vi "LoadWave.vi"(10 "Variables":T3={"Number of rings"=1, "sound spd (cm/s)"=150000, "z span (cm)"=4.0, "z steps"=20, "y spacing (cm)"=0.01, "y steps"=50, "time step (s)"=1e-08, "z"=0.0, "y"=0.0, "ref delay"=0.0, "freq (MHz)"=4.71, "cycles"=300.0} {"freq (MHz)" format="%.2f"; "z span (cm)" format="%.2f"; "y" format="%.2f"; "ref delay" format="%.2f"; "y spacing (cm)" format="%.2f"; "z" format="%.2f"; "time step (s)" format="%.2e"}, 11 "Wave Source":T1={"Load Wave File"=FALSE, "file path"=path "F:/PVDFXducer/FiveRing/5Ring5/83micH/R1quartz.txt", "Up sample fac"=1}) -> (3 "Waveform Graph":dbl[](graph))   [LabVIEW 2022 SP3]
uses:
  <vilib>/Analysis/4window.llb/Hamming Window (DBL).vi
  <vilib>/Analysis/4window.llb/AllCosWindow (DBL).vi
  <vilib>/Utility/file.llb/Read From Spreadsheet File (DBL).vi
  <vilib>/Analysis/2dsp.llb/Rational Resample (single channel, DBL).vi
  <vilib>/Analysis/NI_AALPro.lvlib
panel:
  out "Spectrum":T2(graph)
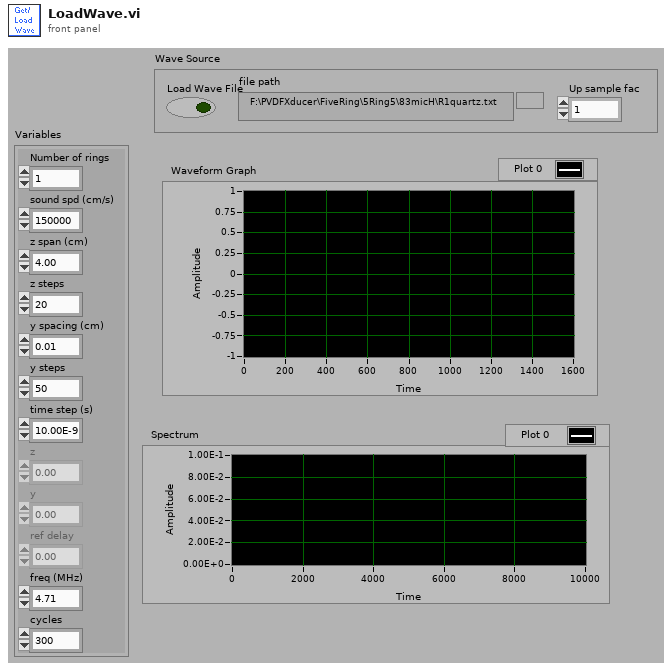
[diagram p1: front panel]
types:
  T1 = cluster{"Load Wave File":bool, "file path":path, "Up sample fac":i32}
  T2 = cluster{i32, "df":dbl, "Power Spectrum (V^2 rms)":dbl[]}
  T3 = cluster{"Number of rings":i32, "sound spd (cm/s)":i32, "z span (cm)":dbl, "z steps":i32, "y spacing (cm)":dbl, "y steps":i32, "time step (s)":sgl, "z":dbl, "y":dbl, "ref delay":dbl, "freq (MHz)":dbl, "cycles":sgl}
  T4 = enum16{"sine", "cosine", "triangle", "square", "sawtooth", "increasing ramp", "decreasing ramp"}
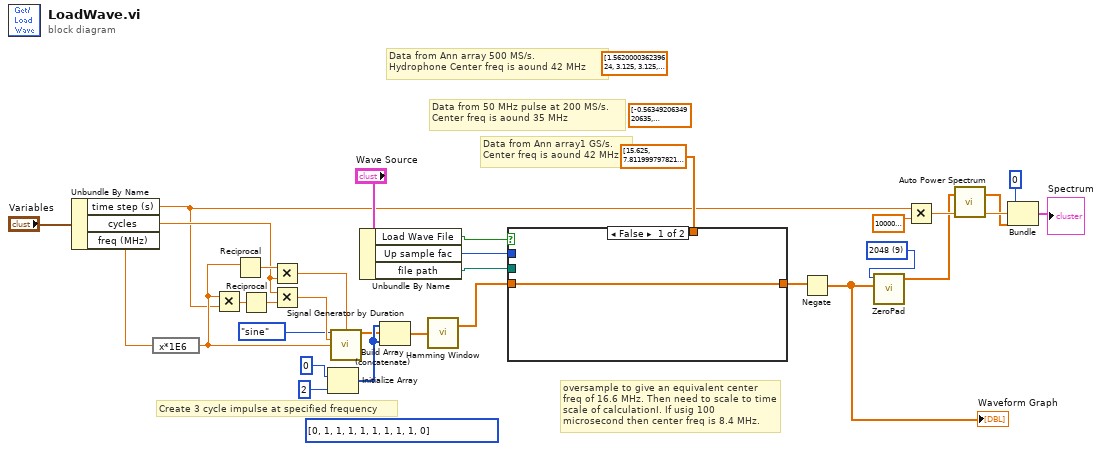
[diagram p0: block diagram]
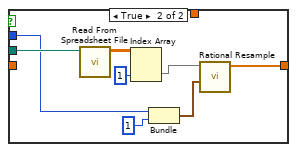
[diagram p2: hidden frame]
diagram:
  w2 = u16 9 items=["next 2^n", "8", "16", "32", "64", "128", "256", "512", "1024", "2048"] ("FFT size")
  (unwired) sgl[] [1.562, 3.125, 3.125, 3.906, 3.125, 1.562, 1.562, 2.344, 3.125, 3.125, 3.125, 3.906, 4.687, 4.687, 5.469, 4.687, 3.125, 1.562, 1.562, 0.781, 1.562, 1.562, 1.562, 3.125, 3.125, 2.344, 1.562, 3.125, 2.344, 0.781, 0.0, 0.0, -0.781, -0.781, 0.0, 1.562, 3.125, 3.125, 3.125, 3.125, 2.344, 1.562, -0.781, -0.781, 0.781, 3.125, 3.125, 3.906, 3.906, 3.906, 4.687, 3.125, 1.562, 1.562, 2.344, 2.344, 2.344, 3.125, 3.906, 3.125, 2.344, 0.781, 0.0, -0.781, 0.781, 0.781, 0.781, 0.781, 0.781, 0.0, 0.0, 0.0, 0.0, 0.0, -0.781, -1.562, -3.125, -3.125, -4.687, -3.906, -7.031, -10.156, -12.5, -16.406, -18.75, -22.656, -24.219, -18.75, -9.375, 7.812, 28.125, 47.656, 65.625, 73.437, 73.437, 66.406, 53.906, 41.406, 27.344, 14.844, 3.906, -5.469, -14.062, -22.656, -25.781, -26.562, -25.0, -24.219, -21.875, -21.875, -25.0, -28.125, -32.812, -37.5, -44.531, -46.875, -43.75, -32.031, -15.625, 3.125, 25.0, 39.062, 47.656, 50.0, 45.312, 35.156, 24.219, 13.281, 4.687, -3.906, -9.375, -12.5, -13.281, -17.187, -17.187, -14.062, -7.812, -3.125, 1.562, 0.781, -0.781, -3.906, -6.25, -8.594, -8.594, -9.375, -7.031, -3.125, 0.0, 4.687, 6.25, 8.594, 8.594, 10.937, 10.156, 10.156, 9.375, 7.812, 4.687, 1.562, -0.781, -2.344, -3.125, -3.906, -3.125, -2.344, -0.781, 1.562, 3.125, 3.125, 1.562, 1.562, 1.562, 1.562, 1.562, 2.344, 3.906, 3.125, 3.125, 3.125, 2.344, 2.344, 0.781, -0.781, 0.0, 3.125, 4.687, 6.25, 5.469, 5.469, 6.25, 6.25, 6.25, 4.687, 6.25, 7.031, 6.25, 6.25, 6.25, 9.375, 9.375, 7.812, 7.031, 7.031, 7.031, 5.469, 5.469, 5.469, 5.469, 5.469, 4.687, 3.125, 3.125, 2.344, 2.344, 1.562, 3.125, 5.469, 5.469, 5.469, 5.469, 5.469, 5.469, 4.687, 3.906, 3.906, 3.125, 3.125, 3.906, 2.344, 1.562, 2.344, 2.344, 3.125, 3.125, 3.125, 3.125, 3.125, 1.562, 0.781, 0.0, 0.781, 0.0] ("first row")
  (unwired) i32[] [0, 1, 1, 1, 1, 1, 1, 1, 1, 0] ("first row")
  (unwired) dbl[] [-0.5634920634920635, -0.6825396825396826, -0.8015873015873016, -0.9920634920634921, -1.1507936507936507, -1.3888888888888888, -1.992063492063492, -4.2063492063492065, -5.888888888888889, 13.023809523809524, 61.32539682539682, 92.83333333333333, 75.10317460317461, 18.126984126984127, -54.93650793650794, -109.60317460317461, -104.22222222222223, 18.134920634920636, 83.33333333333333, 27.27777777777778, -42.19047619047619, -45.63492063492063, 10.15079365079365, 49.05555555555556, 28.19047619047619, -5.658730158730159, -15.261904761904763, -4.4603174603174605, 7.984126984126984, 10.682539682539682, 5.809523809523809, -0.03968253968253968, -2.515873015873016, -1.4841269841269842, 1.0396825396825398, 2.0555555555555554, 0.9523809523809523, -0.6031746031746031, -1.007936507936508, -0.3968253968253968, 0.14285714285714285] ("Array")
  # "Create 3 cycle impulse at specified frequency"
  # "Data from Ann array 500 MS/s.\nHydrophone Center freq is aound 42 MHz"
  # "Data from Ann array1 GS/s.\nCenter freq is aound 42 MHz"
  # "oversample to give an equivalent center freq of 16.6 MHz. Then need to scale to time scale of calculationI. If usig 100 microsecond then center freq is 8.4 MHz."
  # "Data from 50 MHz pulse at 200 MS/s.\nCenter freq is aound 35 MHz"
  n1 = Unbundle By Name("Variables") -> ("time step (s)"=w5:sgl, "cycles"=w19:sgl, "freq (MHz)"=w20:dbl)
  n2 = expression code="x*1E6"(w20) -> (w23:dbl)
  n3 = Multiply(x=w23, y=w5) -> (x*y=w27:dbl)
  n4 = Reciprocal(x=w23) -> (1/x=w22:dbl)
  n5 = Reciprocal(x=w27) -> (1/x=w24:dbl)
  n6 = Multiply(x=w22, y=w19) -> (x*y=w21:dbl)
  n7 = Multiply(x=w19, y=w24) -> (x*y=w26:dbl)
  n8 = Initialize Array(0, 2) -> (w16:i32[])
  n9 = call <vilib>:"Signal Generator by Duration.vi"("signal type"=T4."sine", "duration"=w21, "# of samples"=w26, "frequency"=w23) -> ("signal"=w15:dbl[])  [unwired: 3 in, 8 out]
  n10 = Unbundle By Name("Wave Source") -> ("Load Wave File"=w11:bool, "Up sample fac"=w10:i32, "file path"=w9:path)
  n11 = Build Array (concatenate)(w16, w15, w16) -> (w8:dbl[])
  n12 = call-poly <vilib>:"Hamming Window.vi"("X"=w8) -> ("Windowed X"=w7:dbl[])  [unwired: 1 out]
  n13 = case shown="False" w11 {
    tunnel: [w33 w35] -> w4
    tunnel: w7 -> [w33 _]
    tunnel: w9 -> [_ w39]
    tunnel: w10 -> [_ w37]
    tunnel: sgl[] [15.625, 7.812, 7.812, 7.812, 0.0, 7.812, 7.812, 0.0, 0.0, 7.812, 7.812, 7.812, 7.812, 7.812, 7.812, 7.812, 7.812, 7.812, 7.812, 15.625, 7.812, 7.812, 7.812, 15.625, 7.812, 7.812, 7.812, 7.812, 7.812, 15.625, 7.812, 7.812, 7.812, 7.812, 7.812, 7.812, 7.812, 0.0, 7.812, 7.812, 7.812, 0.0, 0.0, 7.812, 7.812, 7.812, 0.0, 7.812, 7.812, 7.812, 7.812, 7.812, 7.812, 7.812, 15.625, 7.812, 7.812, 7.812, 7.812, 7.812, 7.812, 7.812, 7.812, 7.812, 7.812, 7.812, 7.812, 7.812, 7.812, 0.0, 7.812, 7.812, 7.812, 15.625, 7.812, 7.812, 7.812, 7.812, 15.625, 7.812, 7.812, 15.625, 7.812, 7.812, 7.812, 15.625, 0.0, 7.812, 15.625, 7.812, 15.625, 7.812, 7.812, 7.812, 7.812, 7.812, 0.0, 7.812, 7.812, 7.812, 7.812, 7.812, 7.812, 7.812, 7.812, 7.812, 7.812, 7.812, 15.625, 7.812, 7.812, 7.812, 7.812, 7.812, 15.625, 7.812, 7.812, 7.812, 7.812, 7.812, 7.812, 7.812, 7.812, 0.0, 7.812, 0.0, 7.812, 7.812, 7.812, 7.812, 7.812, 7.812, 7.812, 7.812, 7.812, 7.812, 7.812, 7.812, 7.812, 7.812, 0.0, 15.625, 0.0, 7.812, 7.812, 7.812, 7.812, 15.625, 15.625, 7.812, 7.812, 7.812, 7.812, 7.812, 7.812, 7.812, 7.812, 7.812, 7.812, 7.812, 7.812, 7.812, 7.812, 7.812, 7.812, 7.812, 7.812, 7.812, 7.812, 7.812, 15.625, 15.625, 7.812, 7.812, 7.812, 7.812, 0.0, 0.0, 0.0, 7.812, 7.812, 7.812, 7.812, 0.0, 7.812, 15.625, 7.812, 7.812, 15.625, 7.812, 15.625, 7.812, 7.812, 7.812, 7.812, 7.812, 7.812, 7.812, 15.625, 7.812, 7.812, 7.812, 7.812, 7.812, 15.625, 7.812, 7.812, 7.812, 7.812, 7.812, 7.812, 7.812, 7.812, 15.625, 7.812, 7.812, 15.625, 7.812, 15.625, 7.812, 7.812, 7.812, 7.812, 7.812, 7.812, 7.812, 15.625, 15.625, 7.812, 7.812, 7.812, 7.812, 7.812, 15.625, 7.812, 7.812, 7.812, 7.812, 7.812, 7.812, 7.812, 7.812, 7.812, 7.812, 0.0, 7.812, 0.0, 0.0, 7.812, 15.625, 7.812, 7.812, 7.812, 7.812, 7.812, 7.812, 7.812, 7.812, 7.812, 7.812, 7.812, 15.625, 7.812, 7.812, 7.812, 7.812, 7.812, 0.0, 7.812, 7.812, 7.812, 7.812, 7.812, 7.812, 0.0, 0.0, 7.812, 7.812, 7.812, 0.0, 7.812, 7.812, 7.812, 7.812, 7.812, 7.812, 7.812, 7.812, 15.625, 7.812, 7.812, 15.625, 7.812, 7.812, 7.812, 7.812, 7.812, 7.812, 0.0, 7.812, 7.812, 7.812, 15.625, 7.812, 7.812, 7.812, 7.812, 7.812, 7.812, 7.812, 7.812, 7.812, 7.812, 15.625, 7.812, 7.812, 7.812, 7.812, 7.812, 0.0, 7.812, 7.812, 7.812, 7.812, 7.812, 7.812, 7.812, 7.812, 7.812, 15.625, 15.625, 7.812, 7.812, 7.812, 0.0, 7.812, 7.812, 7.812, 7.812, 7.812, 7.812, 7.812, 0.0, 7.812, 7.812, 7.812, 7.812, 7.812, 7.812, 7.812, 0.0, 7.812, 0.0, 7.812, 15.625, 7.812, 7.812, 7.812, 0.0, 7.812, 7.812, 7.812, 15.625, 7.812, 15.625, 7.812, 7.812, 7.812, 0.0, 0.0, 0.0, 7.812, 7.812, 7.812, 7.812, 7.812, 0.0, 0.0, 0.0, -7.812, -15.625, -23.437, -31.25, -39.062, -46.875, -39.062, -31.25, -7.812, 31.25, 78.125, 132.812, 203.125, 257.812, 296.875, 328.125, 335.937, 304.687, 265.625, 179.687, 78.125, -31.25, -140.625, -257.812, -343.75, -421.875, -460.937, -484.375, -484.375, -468.75, -437.5, -406.25, -359.375, -289.062, -210.937, -93.75, 46.875, 210.937, 390.625, 562.5, 718.75, 812.5, 867.187, 851.562, 789.062, 664.062, 468.75, 250.0, 23.437, -210.937, -414.062, -578.125, -687.5, -742.187, -750.0, -703.125, -593.75, -484.375, -359.375, -218.75, -93.75, 31.25, 164.062, 281.25, 390.625, 468.75, 515.625, 515.625, 484.375, 421.875, 320.312, 210.937, 85.937, -39.062, -140.625, -218.75, -273.437, -304.687, -312.5, -296.875, -257.812, -218.75, -164.062, -101.562, -46.875, 0.0, 62.5, 109.375, 156.25, 187.5, 218.75, 218.75, 210.937, 195.312, 164.062, 132.812, 93.75, 54.687, 23.437, -7.812, -39.062, -54.687, -62.5, -70.312, -70.312, -62.5, -54.687, -31.25, -15.625, 0.0, 15.625, 39.062, 54.687, 62.5, 78.125, 85.937, 85.937, 93.75, 78.125, 78.125, 62.5, 46.875, 39.062, 23.437, 7.812, -7.812, -7.812, -15.625, -23.437, -15.625, -23.437, -23.437, -7.812, -15.625, -7.812, 7.812, 7.812, 7.812, 15.625, 15.625, 23.437, 31.25, 23.437, 15.625, 15.625, 15.625, 7.812, 7.812, 0.0, 0.0, 0.0, -7.812, -7.812, -7.812, 0.0, -7.812, -7.812, 0.0, 0.0, -7.812, 0.0, 0.0, 0.0, 0.0, -7.812, 7.812, 0.0, 0.0, 0.0, 0.0, 0.0, 0.0, 0.0, -7.812, 0.0, -7.812, -7.812, -7.812, -7.812, -7.812, 0.0, -7.812, 0.0, -15.625, 0.0, 0.0, 0.0, 0.0, -7.812, -7.812, -7.812, -7.812, -7.812, -7.812, 0.0, 0.0, -7.812, -7.812, 0.0, 0.0, 0.0, 0.0, 0.0, 7.812, 0.0, 0.0, 7.812, 0.0, 7.812, 7.812, 0.0, 0.0, 0.0, 7.812, 0.0, 7.812, 0.0, 0.0, 7.812, 0.0, 7.812, 15.625, 7.812, 7.812, 7.812, 7.812, 15.625, 15.625, 7.812, 15.625, 15.625, 7.812, 15.625, 7.812, 15.625, 7.812, 7.812, 7.812, 15.625, 15.625, 15.625, 15.625, 15.625, 15.625, 15.625, 15.625, 15.625, 7.812, 7.812, 15.625, 15.625, 15.625, 15.625, 15.625, 15.625, 15.625, 15.625, 15.625, 15.625, 15.625, 15.625, 15.625, 15.625, 15.625, 23.437, 15.625, 15.625, 23.437, 15.625, 23.437, 15.625, 15.625, 23.437, 15.625, 15.625, 23.437, 15.625, 15.625, 15.625, 15.625, 15.625, 15.625, 23.437, 15.625, 15.625, 23.437, 15.625, 15.625, 15.625, 15.625, 15.625, 15.625, 15.625, 15.625, 15.625, 15.625, 15.625, 15.625, 15.625, 15.625, 15.625, 15.625, 23.437, 15.625, 23.437, 15.625, 15.625, 15.625, 7.812, 15.625, 15.625, 15.625, 15.625, 7.812, 15.625, 15.625, 7.812, 15.625, 15.625, 15.625, 15.625, 7.812, 7.812, 15.625, 7.812, 15.625, 15.625, 15.625, 7.812, 15.625, 7.812, 7.812, 15.625, 7.812, 7.812, 15.625, 15.625, 7.812, 7.812, 7.812, 7.812, 7.812, 15.625, 0.0, 7.812, 7.812, 7.812, 7.812, 7.812, 0.0, 0.0, 7.812, 7.812, 0.0, 0.0, 0.0, 0.0, 0.0, 7.812, 7.812, 0.0, 7.812, 0.0, 0.0, 7.812, 7.812, 7.812, 7.812, 7.812, 0.0, 0.0, 0.0, 7.812, 7.812, 0.0, 0.0, 7.812, 0.0, 7.812, 0.0, 0.0, 7.812, 0.0, 7.812, 7.812, 0.0, 0.0, 7.812, 0.0, 0.0, 7.812, 0.0, 0.0, 0.0, 0.0, 0.0, 0.0, 7.812, 0.0, 0.0, 0.0, 0.0, 0.0, 7.812, 0.0, 7.812, 7.812, 0.0, 7.812, 0.0, 0.0, 7.812, 7.812, 7.812, 0.0, 7.812, 0.0, 7.812, 0.0, 7.812, 0.0, 0.0, 7.812, 7.812, 0.0, 7.812, 0.0, 0.0, 0.0, 7.812, 0.0, 0.0, 0.0, 0.0, 7.812, 7.812, 7.812, 0.0, 7.812, 0.0, 7.812, 0.0, 0.0, 0.0, 7.812, 7.812, 7.812, 7.812, 0.0, 7.812, 7.812, 7.812, 15.625, 7.812, 7.812, 7.812, 7.812, 7.812, 7.812, 7.812, 7.812, 7.812, 7.812, 15.625, 7.812, 15.625, 7.812, 7.812, 7.812, 7.812, 15.625, 7.812, 7.812, 7.812, 15.625, 15.625, 15.625, 7.812, 15.625, 7.812, 15.625, 15.625, 15.625, 15.625, 7.812, 7.812, 7.812, 15.625, 7.812, 15.625, 15.625, 7.812, 15.625, 7.812, 7.812, 15.625, 15.625, 15.625, 7.812, 7.812, 7.812, 15.625, 15.625, 15.625, 15.625, 15.625, 15.625, 15.625, 15.625, 15.625, 7.812, 15.625, 15.625, 15.625, 15.625, 15.625, 15.625, 7.812, 15.625, 7.812, 7.812, 15.625, 7.812, 7.812, 15.625, 7.812, 7.812, 15.625, 15.625, 15.625, 15.625, 7.812, 7.812, 15.625, 7.812, 7.812, 15.625, 7.812, 15.625, 15.625, 7.812, 15.625, 15.625, 15.625, 15.625, 15.625, 15.625, 15.625, 15.625, 15.625, 7.812, 15.625, 15.625, 15.625, 15.625, 7.812, 7.812, 7.812, 7.812, 7.812, 15.625, 7.812, 7.812, 15.625, 7.812, 15.625, 7.812, 15.625, 15.625, 15.625, 15.625, 7.812, 15.625, 7.812, 7.812, 7.812, 7.812, 7.812, 7.812, 15.625, 15.625, 7.812, 7.812, 7.812, 7.812, 7.812, 7.812, 7.812, 7.812, 7.812, 7.812, 7.812, 7.812, 7.812, 15.625, 7.812, 7.812, 7.812, 7.812, 7.812, 7.812, 0.0, 7.812, 7.812, 0.0, 0.0, 7.812, 7.812, 7.812, 7.812, 7.812, 7.812, 7.812, 7.812, 7.812, 7.812, 7.812, 0.0, 7.812, 7.812, 7.812, 0.0, 7.812, 7.812, 7.812, 0.0, 7.812, 0.0, 7.812, 7.812, 0.0, 0.0, 7.812, 7.812, 7.812, 0.0, 0.0, 7.812, 7.812, 7.812, 0.0, 7.812, 0.0, 0.0, 0.0] ("first row") -> [_ _]
    frame False {
    }
    frame True {
      n14 = call-poly <vilib>:"Read From Spreadsheet File.vi"("file path (dialog if empty)"=w39) -> ("all rows"=w40:dbl[][])  [unwired: 3 in, 7 out]
      n15 = Index Array(array=w40, index (col)=1) -> (element=w34:dbl[])  [unwired: 1 in]
      n16 = Bundle("Up sample fac"=w37, 1) -> (w36:cluster{"Up sample fac":i32, i32})  [unwired: 1 in]
      n17 = call-poly <vilib>:"Rational Resample.vi"("resample factor"=w36, "X"=w34) -> ("Y"=w35:dbl[])  [unwired: 7 in, 2 out]
    }
  }
  n18 = Negate(x=w4) -> (-x=w1:dbl[])
  "Waveform Graph" <- w1
  n19 = call "ZeroPad.vi"("Input Array"=w1, "FFT size"=w2) -> ("Ouput Array"=w3:dbl[])  [unwired: 4 out]
  n20 = Multiply(x=w5, y=1000000.0) -> (x*y=w32:dbl)
  n21 = call <vilib>:"Auto Power Spectrum.vi"("dt"=w32, "Signal (V)"=w3) -> ("df"=w31:dbl, "Power Spectrum (V^2 rms)"=w30:dbl[])
  n22 = Bundle(0, "df"=w31, "Power Spectrum (V^2 rms)"=w30) -> (→"Spectrum":T2)  [unwired: 1 out]
